vi "MB Serial Receive.vi"(7 "Serial Parameters":T1 {"Slave Address" format="%.0x"}, 8 "error in (no error)":errorcluster, 9 "Timeout":u32=10000, 11 "VISA resource name":refnum<visa-resource-name>) -> (0 "error out":errorcluster, 1 "Exception Code":u8 format="%.0x", 2 "Modbus Data Unit":T2={"Function Code"=1, "Data"=[]} {"Function Code" items=["Read Coils"=1, "Read Discrete Inputs"=2, "Read Holding Registers"=3, "Read Input Registers"=4, "Write Single Coil"=5, "Write Single Register"=6, "Read Exception Status"=7, "Write Multiple Coils"=15, "Write Multiple Registers"=16]; "Data" format="%.0x"}, 3 "VISA resource name out":refnum<visa-resource-name>)   [LabVIEW 2012]
uses:
  MB Modbus Data Unit.ctl
panel:
  # "VI Name: MB Serial Receive.vi\nPurpose: Reads a Modbus message.\nReentrant."
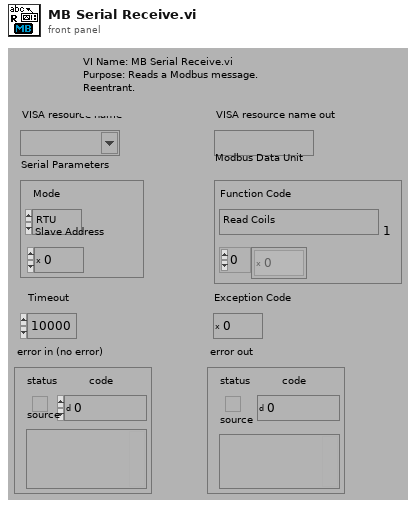
[diagram p1: front panel]
types:
  T1 = cluster{"Mode":enum16{"RTU", "ASCII"}, "Slave Address":u8}
  T2 = typedef "MB Modbus Data Unit.ctl" = cluster{"Function Code":u8, "Data":u8[]}
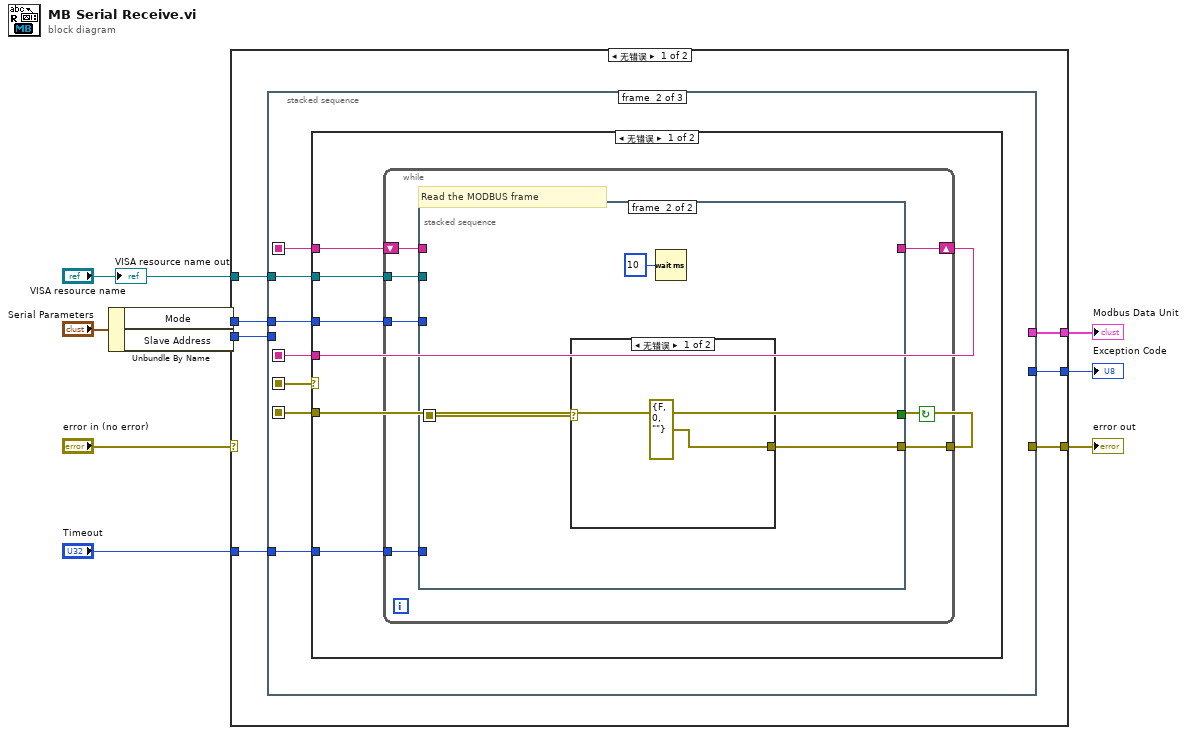
[diagram p0: block diagram]
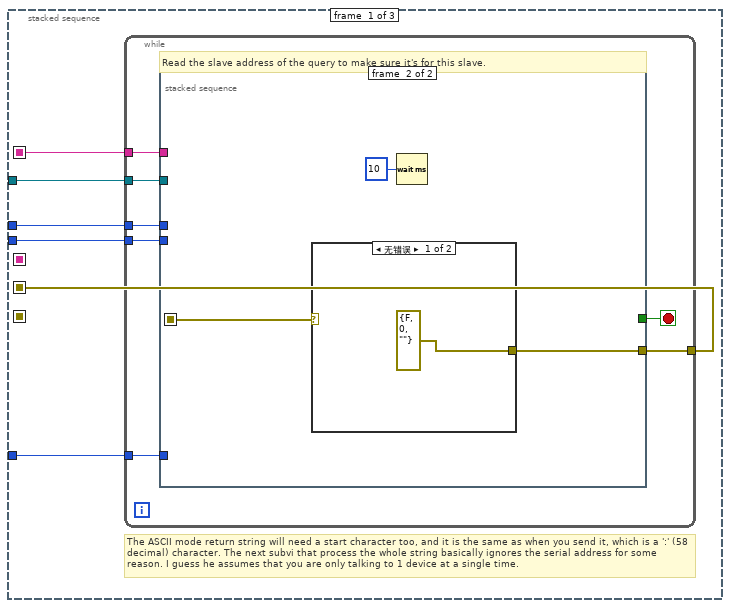
[diagram p2: hidden frame]
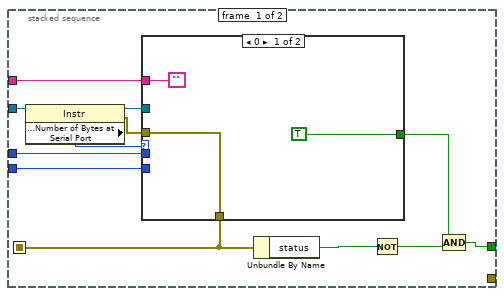
[diagram p3: hidden frame]
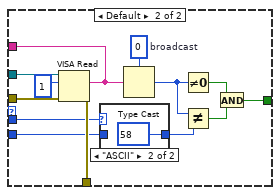
[diagram p4: hidden frame]
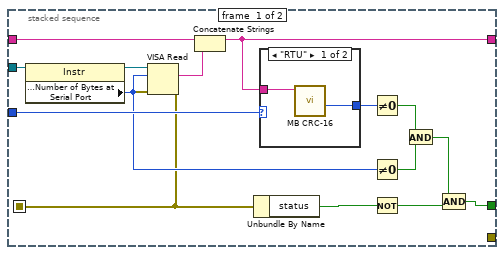
[diagram p7: hidden frame]
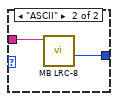
[diagram p8: hidden frame]
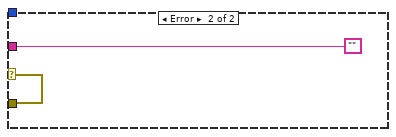
[diagram p10: hidden frame]
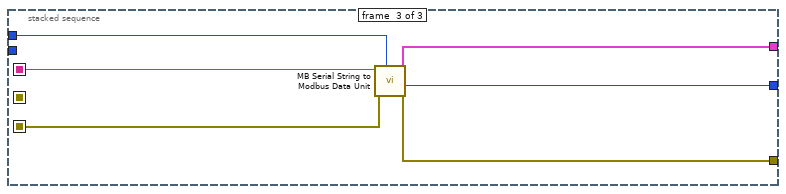
[diagram p11: hidden frame]
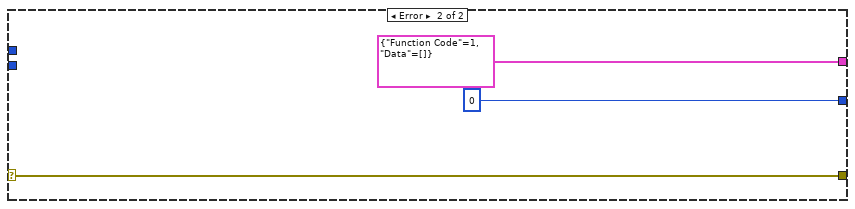
[diagram p12: hidden frame]
diagram:
  n1 = Unbundle By Name("Serial Parameters") -> ("Mode"=w2:enum16{"RTU", "ASCII"}, "Slave Address"=w1:u8)
  n2 = case shown="无错误" "error in (no error)" {
    selector: "error in (no error)" -> [_ w120]
    tunnel: "VISA resource name" -> [w16 _]
    tunnel: w2 -> [w15 _]
    tunnel: [w14 w120] -> w8
    tunnel: [w13 u8 0 ("Exception Code")] -> w6
    tunnel: [w12 T2 {"Function Code"=1, "Data"=[]} ("MODBUS Data Unit")] -> w5
    tunnel: "Timeout" -> [w11 _]
    tunnel: w1 -> [w10 _]
    frame No Error {
      n3 = stacked-sequence {
        seq-local: [_ w69 _] -> [_ _ w115]
        seq-local: [w21 _ _] -> [_ w65 _]
        seq-local: [w19 _ _] -> [_ w67 _]
        seq-local: [_ w66 _] -> [_ _ w112]
        tunnel: w16 -> [w22 w71 _]
        tunnel: w15 -> [w17 w70 w117]
        tunnel: [_ _ w116] -> w14
        tunnel: [_ _ w114] -> w13
        tunnel: [_ _ w113] -> w12
        tunnel: w11 -> [w20 w68 _]
        tunnel: w10 -> [w18 _ _]
        frame #0 {
          # "The ASCII mode return string will need a start character too, and it is the same as when you send it, which is a ':' (58 decimal) character. The next subvi that process the whole string basically ignores the serial address for some reason. I guess he assumes that you are only talking to 1 device at a single time."
          n4 = while {
            tunnel: w22 -> [w28]
            tunnel: [w27] -> w21
            tunnel: w20 -> [w26]
            tunnel: [w25] -> w19
            tunnel: w18 -> [w24]
            tunnel: w17 -> [w23]
            stop <- w29 stop-if-true
            # "Read the slave address of the query to make sure it's for this slave."
            n5 = stacked-sequence {
              seq-local: [w35 _] -> [_ w61]
              tunnel: [w41 _] -> w29
              tunnel: w28 -> [w40 _]
              tunnel: [_ w60] -> w27
              tunnel: w26 -> [_ _]
              tunnel: [w34 _] -> w25
              tunnel: w24 -> [w31 _]
              tunnel: w23 -> [w30 _]
              frame #0 {
                n6 = property class="Instr"(reference=w40) -> (reference out=w39:refnum<visa-resource-name>, error out=w38:errorcluster, "Serial Settings:Number of Bytes at Serial Port"=w33:u32)  [unwired: 1 in]
                n7 = case shown="0" w33 {
                  tunnel: w39 -> [_ w57]
                  tunnel: w38 -> [w43 w56]
                  tunnel: [w43 w55] -> w35
                  tunnel: ["" w53] -> w34
                  tunnel: [TRUE w48] -> w32
                  tunnel: w31 -> [_ w47]
                  tunnel: w30 -> [_ w45]
                  frame 0 {
                  }
                  frame Default {
                    w52 = u8 0  # broadcast
                    n8 = VISA Read(VISA resource name=w57, byte count=u32 1, error in (no error)=w56) -> (read buffer=w53:string, error out=w55:errorcluster)  [unwired: 2 out]
                    n9 = case shown="\"ASCII\"" w45 {
                      tunnel: w47 -> [w58 _]
                      tunnel: [w58 u8 58 ("Slave Address")] -> w46
                      frame "RTU", Default {
                      }
                      frame "ASCII" {
                      }
                    }
                    n10 = Type Cast(type=w52, x=w53) -> (*(type *) &x=w51:u8)
                    n11 = Not Equal To 0?(x=w51) -> (x != 0?=w50:bool)
                    n12 = Not Equal?(x=w51, y=w46) -> (x != y?=w49:bool)
                    n13 = And(x=w50, y=w49) -> (x .and. y?=w48:bool)
                  }
                }
                n14 = Unbundle By Name(w35) -> ("status"=w37:bool)
                n15 = Not(x=w37) -> (.not. x?=w36:bool)
                n16 = Compound Arithmetic op=AND(w32, w36) -> (w41:bool)
              }
              frame #1 {
                n17 = case shown="无错误" w61 {
                  selector: w61 -> [_ w64]
                  tunnel: [errorcluster {"status"=FALSE, "code"=0, "source"=""} ("error out") w64] -> w60
                  frame No Error {
                  }
                  frame Error {
                  }
                }
                n18 = Wait (ms)(milliseconds to wait=u32 10) -> ()  [unwired: 1 out]
              }
            }
          }
        }
        frame #1 {
          n19 = case shown="无错误" w65 {
            selector: w65 -> [_ w111]
            tunnel: w71 -> [w77 _]
            tunnel: w70 -> [w76 _]
            tunnel: [w75 ""] -> w69
            tunnel: w68 -> [w74 _]
            tunnel: w67 -> [w73 _]
            tunnel: [w72 w111] -> w66
            frame No Error {
              n20 = while {
                tunnel: w76 -> [w83]
                shift-left: w73 -> [w81]
                shift-right: [w78] -> w75
                tunnel: w77 -> [w82]
                tunnel: [w80] -> w72
                tunnel: w74 -> [w79]
                stop <- w84 continue-if-true
                # "Read the MODBUS frame"
                n21 = stacked-sequence {
                  seq-local: [w85 _] -> [_ w106]
                  tunnel: [w100 _] -> w84
                  tunnel: w83 -> [w99 _]
                  tunnel: w82 -> [w94 _]
                  tunnel: w81 -> [w90 _]
                  tunnel: [w88 _] -> w78
                  tunnel: [_ w105] -> w80
                  tunnel: w79 -> [_ _]
                  frame #0 {
                    n22 = property class="Instr"(reference=w94) -> (reference out=w93:refnum<visa-resource-name>, error out=w91:errorcluster, "Serial Settings:Number of Bytes at Serial Port"=w92:u32)  [unwired: 1 in]
                    n23 = VISA Read(VISA resource name=w93, byte count=w92, error in (no error)=w91) -> (read buffer=w89:string, error out=w85:errorcluster)  [unwired: 2 out]
                    n24 = Concatenate Strings(w90, w89) -> (w88:string)
                    n25 = Unbundle By Name(w85) -> ("status"=w87:bool)
                    n26 = case shown="\"RTU\"" w99 {
                      tunnel: w88 -> [w102 w104]
                      tunnel: [w101 w103] -> w98
                      frame "RTU" {
                        n27 = call "MB CRC-16.vi"("String"=w102) -> ("CRC-16"=w101:u8)  [unwired: 10 out]
                      }
                      frame "ASCII" {
                        n28 = call "MB LRC-8.vi"("String"=w104) -> ("LRC-8"=w103:u8)  [unwired: 10 out]
                      }
                    }
                    n29 = Not Equal To 0?(x=w98) -> (x != 0?=w97:bool)
                    n30 = Not Equal To 0?(x=w92) -> (x != 0?=w95:bool)
                    n31 = Not(x=w87) -> (.not. x?=w86:bool)
                    n32 = And(x=w97, y=w95) -> (x .and. y?=w96:bool)
                    n33 = Compound Arithmetic op=AND(w96, w86) -> (w100:bool)
                  }
                  frame #1 {
                    n34 = case shown="无错误" w106 {
                      selector: w106 -> [_ w109]
                      tunnel: [errorcluster {"status"=FALSE, "code"=0, "source"=""} ("error out") w109] -> w105
                      frame No Error {
                      }
                      frame Error {
                      }
                    }
                    n35 = Wait (ms)(milliseconds to wait=u32 10) -> ()  [unwired: 1 out]
                  }
                }
              }
            }
            frame Error {
            }
          }
        }
        frame #2 {
          n36 = call "MB Serial String to Modbus Data Unit.vi"("Mode"=w117, "error in (no error)"=w112, "String"=w115) -> ("error out"=w116:errorcluster, "Exception Code"=w114:u8, "Modbus Data Unit"=w113:T2)  [unwired: 1 in, 5 out]
        }
      }
    }
    frame Error {
    }
  }
  "error out" <- w8
  "Exception Code" <- w6
  "Modbus Data Unit" <- w5
  "VISA resource name out" <- "VISA resource name"
